vi "Redraw Points and Path.vi"(8 "error in (no error)":errorcluster, 11 "GarphView in":refnum<class "GarphView.lvclass">) -> (0 "error out":errorcluster, 3 "GarphView out":refnum<class "GarphView.lvclass">)   [LabVIEW 2020, in "GarphView.lvlib" / "GarphView.lvclass"]
uses:
  GarphView.lvclass
  Range Arrows.ctl
  <vilib>/Utility/miscctls.llb/LVPoint32TypeDef.ctl
  Coords Point.ctl
  GarphView.lvclass/GarphView.ctl
  <vilib>/gpm_packages/@cs/lookup-table/Source/LookupTable/LookupTable.lvclass/LookupTable.ctl
  7c259eef-699e-4564-901b-348da09fba39.vi
  3b04f13f-ec94-4820-b9ee-e210a47742eb.vi
  <vilib>/gpm_packages/@cs/lookup-table/Source/LookupTable/Read Table Reference.vi
  <vilib>/gpm_packages/@cs/lookup-table/Source/LookupTable/LookupTable.lvclass
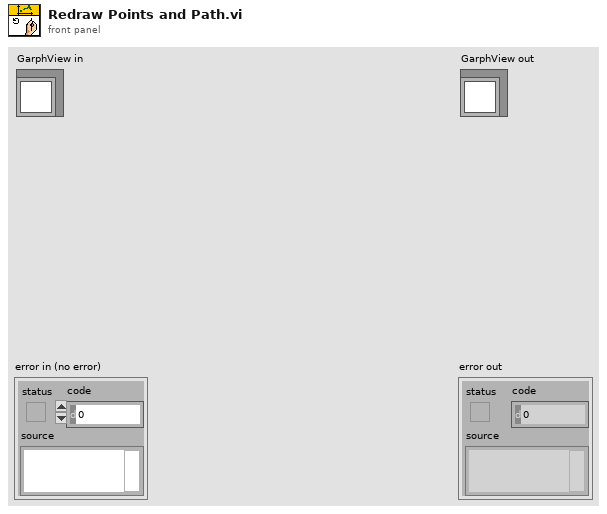
[diagram p1: front panel]
types:
  T1 = typedef "GarphView.lvlib/GarphView.lvclass/Coords Point.ctl" = cluster{"XY":cluster{"X":dbl, "Y":dbl}, "Name":string}
  T2 = typedef "GarphView.lvlib/GarphView.lvclass/Range Arrows.ctl" = cluster{"end Coords":T3, "Start Coords":T3}
  T3 = typedef "LVPoint32TypeDef.ctl" = cluster{"Horizontal":i32, "Vertical":i32}
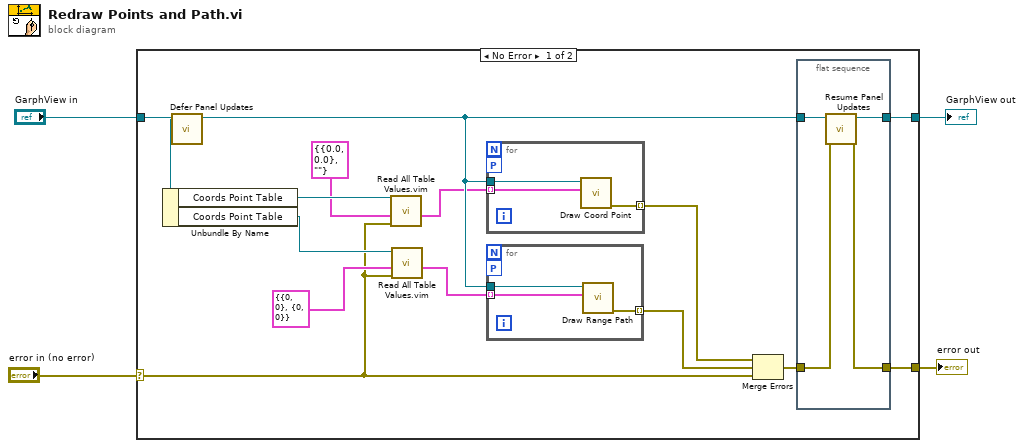
[diagram p0: block diagram]
diagram:
  n1 = case shown="No Error" "error in (no error)" {
    selector: "error in (no error)" -> [w5 w30]
    tunnel: [w14 w30] -> w3
    tunnel: [w13 w29] -> w1
    tunnel: "GarphView in" -> [w18 w29]
    frame No Error {
      n2 = call-dynamic "Defer Panel Updates.vi"("IViewable In"=w18) -> ("IViewable Out"=w12:refnum<class "GarphView.lvclass">)  [unwired: 9 in, 1 out]
      n3 = Unbundle By Name(w12) -> ("Coords Point Table"=w11:refnum<data-value>, "Coords Point Table"=w10:refnum<data-value>)
      n4 = call "Read All Table Values.vim"("error in (no error)"=w5, "Type (All)"=T1 {"XY"={"X"=0.0, "Y"=0.0}, "Name"=""} ("Coords Point"), "LookupTable Reference"=w11) -> ("Values"=w7:T1[])  [unwired: 5 in, 3 out]
      n5 = call "Read All Table Values.vim"("error in (no error)"=w5, "Type (All)"=T2 {"end Coords"={"Horizontal"=0, "Vertical"=0}, "Start Coords"={"Horizontal"=0, "Vertical"=0}} ("Range Arrows"), "LookupTable Reference"=w10) -> ("Values"=w6:T2[])  [unwired: 5 in, 3 out]
      n6 = for {
        tunnel: w12 -> [w28]
        tunnel: [w27] -> w16 mode=indexing
        workers-P: _ -> [_]
        tunnel: w7 -> [w26] mode=indexing
        n7 = call-dynamic "Draw Coord Point.vi"("XY"=w26, "GarphView in"=w28) -> ("error out"=w27:errorcluster)  [unwired: 8 in, 1 out]
      }
      n8 = for {
        tunnel: w12 -> [w25]
        tunnel: [w24] -> w17 mode=indexing
        workers-P: _ -> [_]
        tunnel: w6 -> [w23] mode=indexing
        n9 = call-dynamic "Draw Range Path.vi"("Range Arrows"=w23, "GarphView in"=w25) -> ("error out"=w24:errorcluster)  [unwired: 8 in, 1 out]
      }
      n10 = Merge Errors(w16, w17, w5) -> (w15:errorcluster)
      n11 = flat-sequence {
        tunnel: w12 -> [w22]
        tunnel: w15 -> [w21]
        tunnel: [w20] -> w14
        tunnel: [w19] -> w13
        frame #0 {
          n12 = call-dynamic "Resume Panel Updates.vi"("error in (no error)"=w21, "IViewable In"=w22) -> ("error out"=w20:errorcluster, "IViewable Out"=w19:refnum<class "GarphView.lvclass">)  [unwired: 8 in]
        }
      }
    }
    frame Error {
    }
  }
  "error out" <- w3
  "GarphView out" <- w1
